vi "Global 1.vi"() -> ()   [LabVIEW 2021]
panel:
  in  "sampling info":cluster{"Fs":dbl, "#s":dbl}={"Fs"=1000.0, "#s"=1000.0} {"Fs" format="%.2p"}
  in  "Waveform":waveform(dbl)
  out "Generating":bool
  in  "Signal":string
  in  "Actual":dbl
  out "Ready":bool
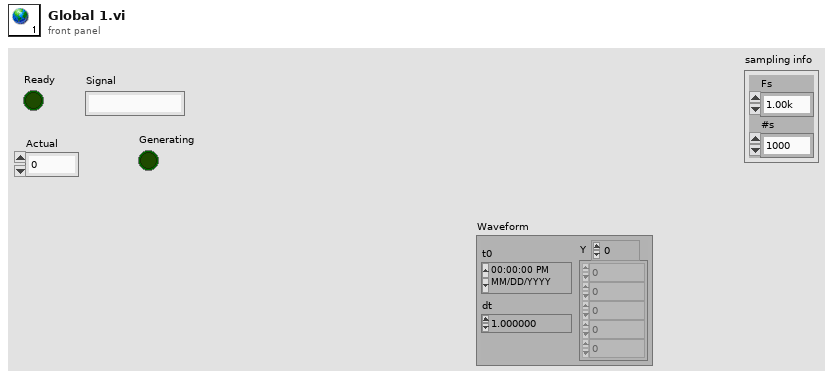
[diagram p1: front panel]
diagram:
